vi "mining_control.vi"() -> ()   [LabVIEW 2015]
panel:
  in  "Boolean":bool
  in  "ACTIVATE\nWINCH":bool
  in  "Winch UP":bool
  in  "Winch DOWN\n(SLOW)":bool
  in  "Winch DOWN":bool
  # "Must turn active button off before activating        a different button"
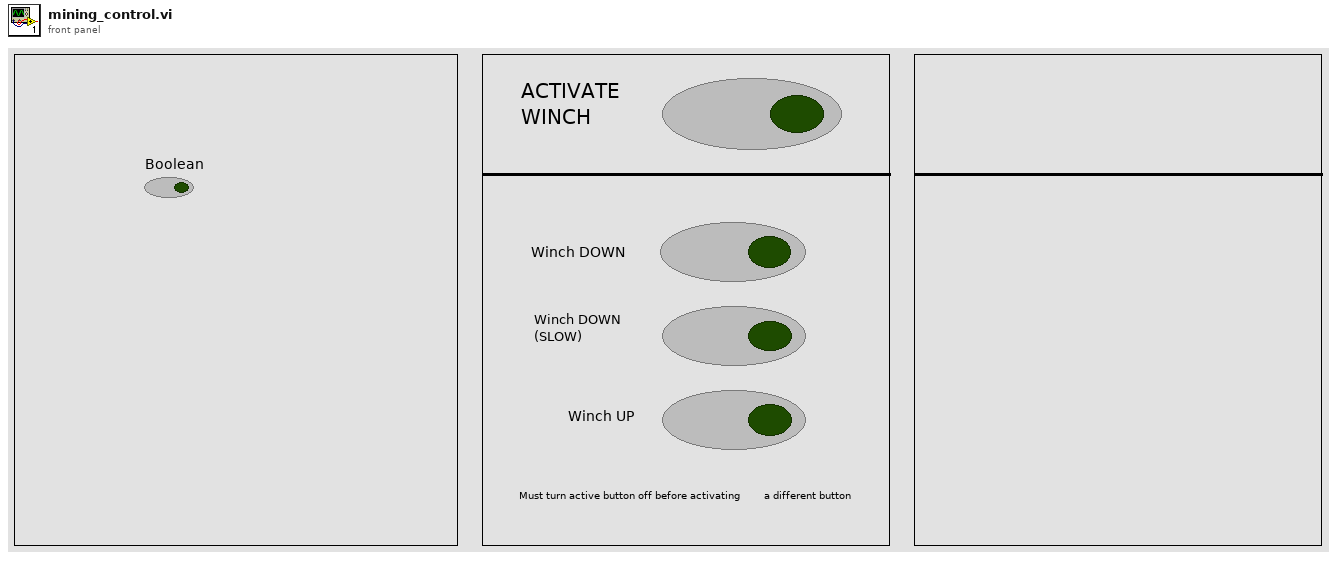
[diagram p1: front panel]
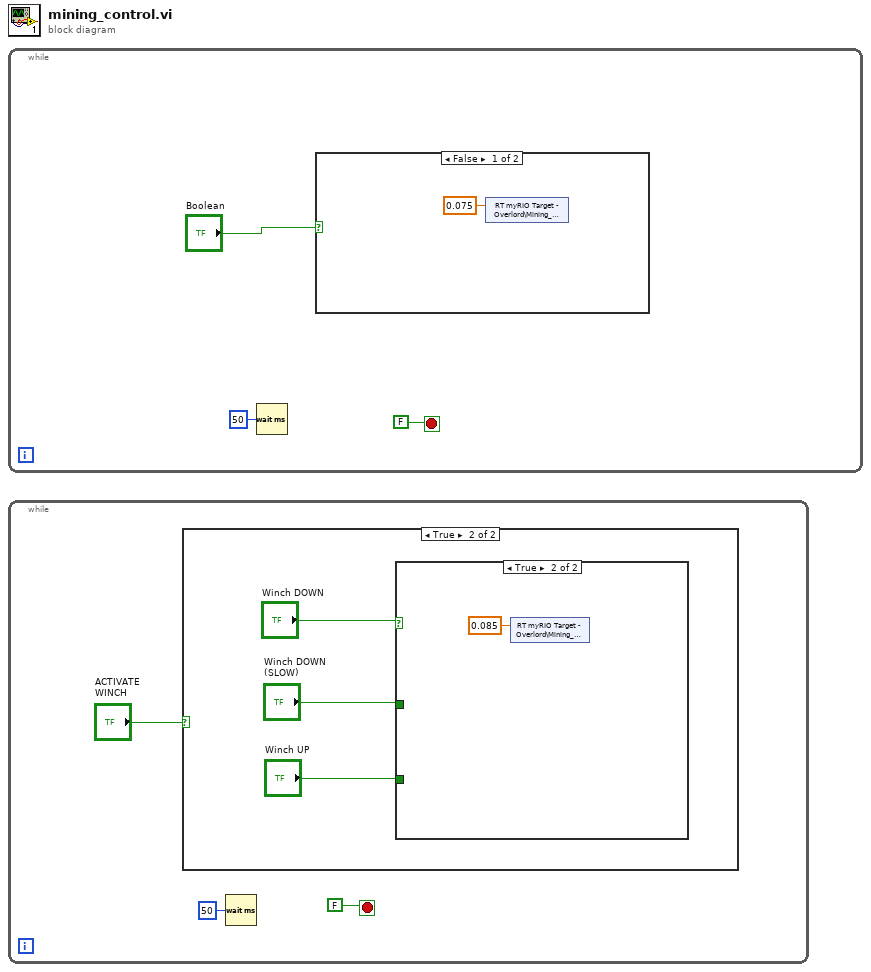
[diagram p0: block diagram]
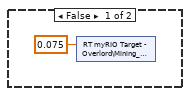
[diagram p2: hidden frame]
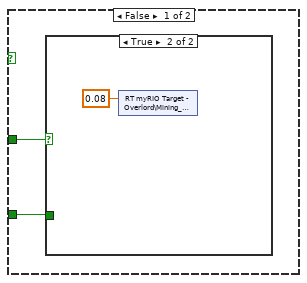
[diagram p3: hidden frame]
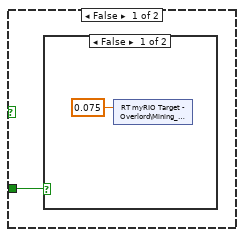
[diagram p4: hidden frame]
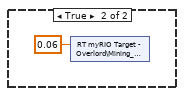
[diagram p5: hidden frame]
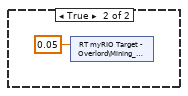
[diagram p6: hidden frame]
diagram:
  n1 = while {
    stop <- FALSE stop-if-true
    n2 = Wait (ms)(milliseconds to wait=u32 50) -> ()  [unwired: 1 out]
    n3 = case shown="False" "Boolean" {
      frame False {
        n4 = shared-variable "RT myRIO Target - Overlord\\Mining_Variables_r0.lvlib\\Scoops"(0.075 ("Scoops")) -> ()  [unwired: 1 in, 1 out]
      }
      frame True {
        n5 = shared-variable "RT myRIO Target - Overlord\\Mining_Variables_r0.lvlib\\Scoops"(0.05 ("Scoops")) -> ()  [unwired: 1 in, 1 out]
      }
    }
  }
  n6 = while {
    stop <- FALSE stop-if-true
    n7 = case shown="True" "ACTIVATE\nWINCH" {
      frame False {
        n8 = shared-variable "RT myRIO Target - Overlord\\Mining_Variables_r0.lvlib\\Winch"(0.075 ("Winch")) -> ()  [unwired: 1 in, 1 out]
      }
      frame True {
        n9 = case shown="True" "Winch DOWN" {
          tunnel: "Winch DOWN\n(SLOW)" -> [w14 _]
          tunnel: "Winch UP" -> [w13 _]
          frame False {
            n10 = case shown="True" w14 {
              tunnel: w13 -> [w15 _]
              frame False {
                n11 = case shown="False" w15 {
                  frame False {
                    n12 = shared-variable "RT myRIO Target - Overlord\\Mining_Variables_r0.lvlib\\Winch"(0.075 ("Winch")) -> ()  [unwired: 1 in, 1 out]
                  }
                  frame True {
                    n13 = shared-variable "RT myRIO Target - Overlord\\Mining_Variables_r0.lvlib\\Winch"(0.06 ("Winch")) -> ()  [unwired: 1 in, 1 out]
                  }
                }
              }
              frame True {
                n14 = shared-variable "RT myRIO Target - Overlord\\Mining_Variables_r0.lvlib\\Winch"(0.08 ("Winch")) -> ()  [unwired: 1 in, 1 out]
              }
            }
          }
          frame True {
            n15 = shared-variable "RT myRIO Target - Overlord\\Mining_Variables_r0.lvlib\\Winch"(0.085 ("Winch")) -> ()  [unwired: 1 in, 1 out]
          }
        }
      }
    }
    n16 = Wait (ms)(milliseconds to wait=u32 50) -> ()  [unwired: 1 out]
  }
